vi "VerifyLicense_bak.vi"() -> ()   [LabVIEW 2015]
panel:
  in  "用户级别":u16(ring) items=["普通用户", "VIP", "SVIP"]
  out "子字符串 2":string
  out "子字符串":string
  out "user":string
  in  "字符串":string
  in  "UID":string
  out "密钥":string
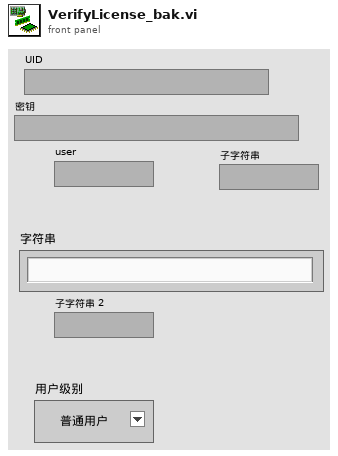
[diagram p1: front panel]
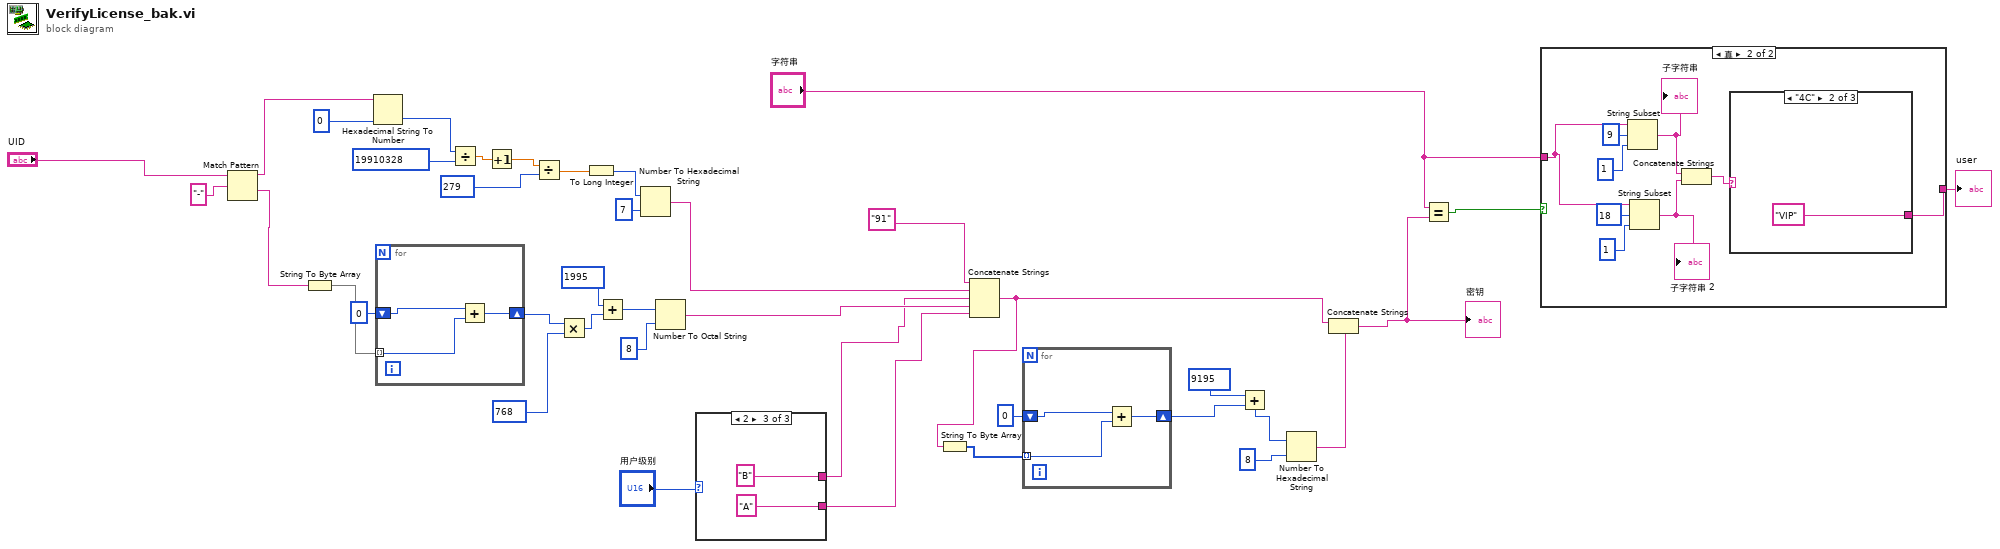
[diagram p0: block diagram]
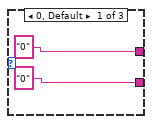
[diagram p2: hidden frame]
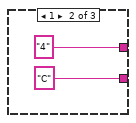
[diagram p3: hidden frame]
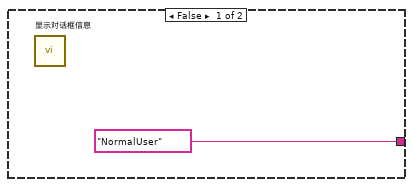
[diagram p4: hidden frame]
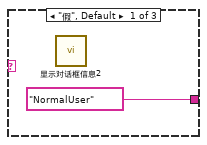
[diagram p5: hidden frame]
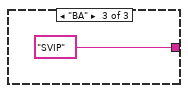
[diagram p6: hidden frame]
diagram:
  n1 = Match Pattern(string="UID", regular expression="-" ("字符串")) -> (before substring=w17:string, after substring=w16:string)  [unwired: 1 in, 2 out]
  n2 = String To Byte Array(string=w16) -> (unsigned byte array=w31:u8[])
  n3 = Hexadecimal String To Number(string=w17, default (0uL)=u64 0 ("默认(0 U32)")) -> (number=w38:u64)  [unwired: 1 in, 1 out]
  n4 = for {
    tunnel: w31 -> [w42] mode=indexing
    shift-right: [w41] -> w29
    shift-left: u8 0 -> [w40]
    n5 = Add(x=w40, y=w42) -> (x+y=w41:u8)
  }
  n6 = Divide(x=w38, y=19910328) -> (x/y=w36:dbl)
  n7 = Increment(x=w36) -> (x+1=w35:dbl)
  n8 = Divide(x=w35, y=279) -> (x/y=w33:dbl)
  n9 = Multiply(x=w29, y=768) -> (x*y=w25:i32)
  n10 = To Long Integer(number=w33) -> (32bit integer=w32:i32)
  n11 = Add(x=1995, y=w25) -> (x+y=w26:i32)
  n12 = Number To Hexadecimal String(1:i16 7 ("宽度(-)"), 2:w32) -> (0:w9:string)
  n13 = Number To Octal String(1:i16 8 ("宽度(-)"), 2:w26) -> (0:w8:string)
  n14 = case shown="2" "用户级别" {
    tunnel: ["0" "4" "B"] -> w2
    tunnel: ["0" "C" "A"] -> w1
    frame 0, Default {
    }
    frame 1 {
    }
    frame 2 {
    }
  }
  n15 = Concatenate Strings("91", w9, w2, w8, w1) -> (w4:string)
  n16 = String To Byte Array(string=w4) -> (unsigned byte array=w20:u8[])
  n17 = for {
    tunnel: w20 -> [w51] mode=indexing
    shift-right: [w50] -> w7
    shift-left: 0 -> [w49]
    n18 = Add(x=w49, y=w51) -> (x+y=w50:i32)
  }
  n19 = Add(x=9195, y=w7) -> (x+y=w6:i32)
  n20 = Number To Hexadecimal String(1:i16 8 ("宽度(-)"), 2:w6) -> (0:w14:string)
  n21 = Concatenate Strings(w4, w14) -> (w13:string)
  "密钥" <- w13
  n22 = Equal?(x="字符串", y=w13) -> (x = y?=w12:bool)
  n23 = case shown="真" w12 {
    tunnel: ["NormalUser" w61] -> w11
    tunnel: "字符串" -> [_ w55]
    frame False {
      n24 = call "显示对话框信息"() -> ()  [unwired: 10 in, 2 out]
    }
    frame True {
      n25 = String Subset(string=w55, offset (0)=9 ("偏移量(0)"), length (rest)=1 ("长度（剩余）")) -> (substring=w58:string)
      "子字符串" <- w58
      n26 = String Subset(string=w55, offset (0)=18 ("偏移量(0)"), length (rest)=1 ("长度（剩余）")) -> (substring=w54:string)
      "子字符串 2" <- w54
      n27 = Concatenate Strings(w58, w54) -> (w53:string)
      n28 = case shown="\"4C\"" w53 {
        tunnel: ["NormalUser" "VIP" "SVIP"] -> w61
        frame "假", Default {
          n29 = call "显示对话框信息2"() -> ()  [unwired: 10 in, 2 out]
        }
        frame "4C" {
        }
        frame "BA" {
        }
      }
    }
  }
  "user" <- w11
